vi "create Chart.vi"(8 "error in (no error)":errorcluster, 10 "Chart Options":T1={"ChartName"="Chart", "BorderDashStyle"=enum."Solid", "Bordercolor"=0, "Title"={"Title"="", "TitleFontSize"=16.0, "fontName"="Arial", "font Color"=0, "Docking"=enum."Top"}, "Legend"={"Docking"=enum."Top", "BorderDashStyle"=enum."NotSet", "BGKcolor"=12763842, "BGKalpha"=81, "Title"="", "TitleSeparator"=enum."None"}} {"Legend"."BGKalpha" scale=0.0..255.0; "Title"."TitleFontSize" min=4.0 max=100.0}, 11 ".NET MSChart":refnum<k24>) -> (0 "error out":errorcluster, 2 ".NET MSChart ChartArea":refnum<k24>, 3 ".NET MSChart":refnum<k24>)   [LabVIEW 2015, in "Graph Extensions MSChart.lvlib"]
uses:
  Graph Extensions MSChart.lvlib
  Controls/Chart.ctl
  Controls/Title.ctl
  Controls/Legend.ctl
  System.Windows.Forms.DataVisualization
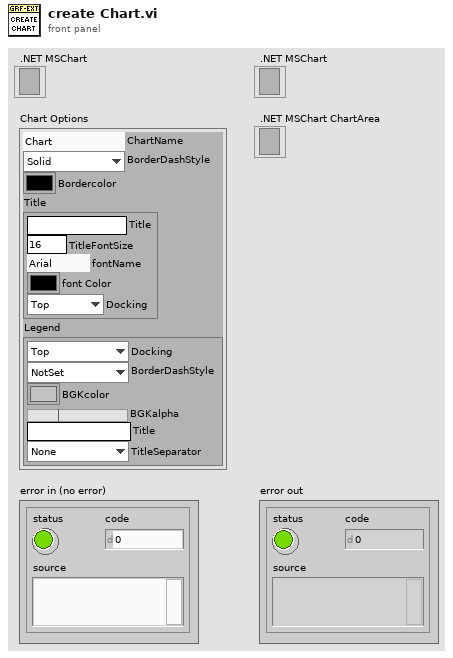
[diagram p1: front panel]
types:
  T1 = typedef "Graph Extensions MSChart.lvlib/Chart.ctl" = cluster{"ChartName":string, "BorderDashStyle":enum16{"NotSet", "Dash", "DashDot", "DashDotDot", "Dot", "Solid"}, "Bordercolor":u32, "Title":T2, "Legend":T3}
  T2 = typedef "Graph Extensions MSChart.lvlib/Title.ctl" = cluster{"Title":string, "TitleFontSize":dbl, "fontName":string, "font Color":u32, "Docking":enum16{"Top", "Right", "Bottom", "Left"}}
  T3 = typedef "Graph Extensions MSChart.lvlib/Legend.ctl" = cluster{"Docking":enum16{"None", "Top", "Right", "Bottom", "Left"}, "BorderDashStyle":enum16{"NotSet", "Dash", "DashDot", "DashDotDot", "Dot", "Solid"}, "BGKcolor":u32, "BGKalpha":u8, "Title":string, "TitleSeparator":enum16{"None", "Line", "ThickLine", "DoubleLine", "DashLine", "DotLine", "GradientLine", "ThickGradientLine"}}
  T4 = enum16{"NotSet", "Dash", "DashDot", "DashDotDot", "Dot", "Solid"}
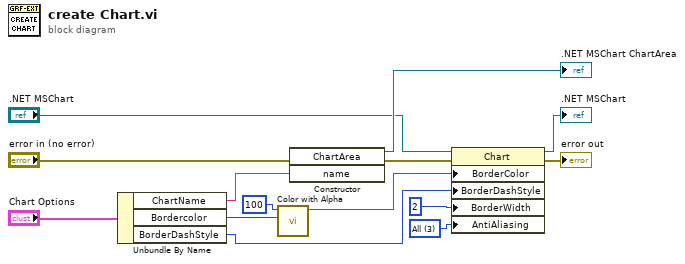
[diagram p0: block diagram]
diagram:
  w11 = 3 items=["None", "Text", "Graphics", "All"] ("AntiAliasing")
  n1 = Unbundle By Name("Chart Options") -> ("ChartName"=w12:string, "Bordercolor"=w7:u32, "BorderDashStyle"=w6:T4)
  n2 = call "Color with Alpha.vi"("Color"=w7, "alpha"=100) -> (".NET color Refnum out"=w10:refnum<k24>)  [unwired: 9 in]
  n3 = constructor class="ChartArea"(error in="error in (no error)", "name"=w12) -> (reference out=→".NET MSChart ChartArea":refnum<k24>, error out=w3:errorcluster)  [unwired: 2 in, 2 out]
  n4 = property class="Chart"(reference=".NET MSChart", error in=w3, "BorderColor"=w10, "BorderDashStyle"=w6, "BorderWidth"=2, "AntiAliasing"=w11) -> (reference out=→".NET MSChart":refnum<k24>, error out=→"error out":errorcluster)
